vi "doDFSM_Error.vi"(0 "NInstrSim":refnum<class "NInstrSim.lvclass">, 3 "DFSM_Internals in":T1, 5 "error in (no error)":errorcluster) -> (14 "dup NInstrSim":refnum<class "NInstrSim.lvclass">, 17 "DFSM_Internals out":T1, 19 "error out":errorcluster)   [LabVIEW 2009, in "HB_Device_Examples.lvlib" / "NInstrSim.lvclass"]
doc: "This VI performs <B>do</B> action of DeviceFSM.Error.\n\n<b>Hint:</b> This is a dynamic dispatch VI to be implemented by child classes."
uses:
  NInstrSim.lvclass
  lib.lib/HGF_LVC/HGF_StateCharts/HGF_DeviceFSM/HGF_DeviceFSM_Internals.ctl
  lib.lib/HGF_LVC/HGF_DeviceBaseClasses/HGF_VISADevice/HGF_VISADevice.lvclass
  lib.lib/HGF_LVC/HGF_DeviceBaseClasses/HGF_DeviceBaseClasses.lvlib
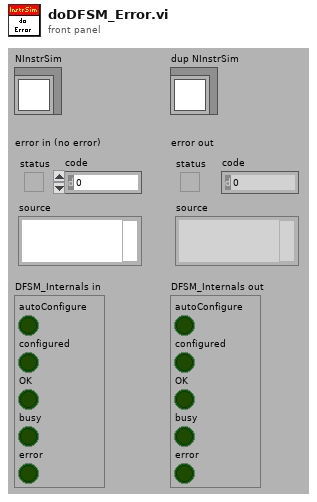
[diagram p1: front panel]
types:
  T1 = typedef "HGF_DeviceBaseClasses.lvlib/HGF_DeviceFSM_Internals.ctl" = cluster{"autoConfigure":bool, "configured":bool, "OK":bool, "busy":bool, "error":bool}
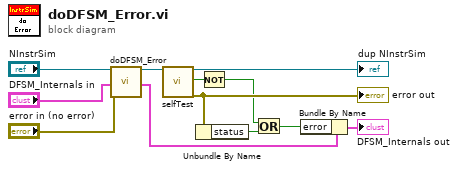
[diagram p0: block diagram]
diagram:
  n1 = call-parent "doDFSM_Error.vi"("HGF_DeviceBase"="NInstrSim", "DFSM_Internals in"="DFSM_Internals in", "error in (no error)"="error in (no error)") -> ("dup HGF_DeviceBase"=w9:refnum<class "NInstrSim.lvclass">, "DFSM_Internals out"=w7:T1)  [unwired: 15 out]
  n2 = call-dynamic "selfTest.vi"("NInstrSim"=w9) -> ("dup NInstrSim"=→"dup NInstrSim":refnum<class "NInstrSim.lvclass">, "passed?"=w5:bool, "error out"=w4:errorcluster)  [unwired: 1 in, 15 out]
  "error out" <- w4
  n3 = Unbundle By Name(w4) -> ("status"=w3:bool)
  n4 = Not(x=w5) -> (.not. x?=w2:bool)
  n5 = Or(x=w2, y=w3) -> (x .or. y?=w1:bool)
  n6 = Bundle By Name(cluster=w7, "error"=w1) -> (→"DFSM_Internals out":T1)
